vi "Emit.vi"(6 "inparameter":variant, 8 "error in (no error)":errorcluster, 9 "parameter":variant, 10 "function":string, 11 "output in":refnum<class "Output.lvclass">) -> (0 "error out":errorcluster, 3 "output out":refnum<class "Output.lvclass">)   [LabVIEW 2015, in "Output.lvclass"]
uses:
  Output.lvclass
  Output.lvclass/Output.ctl
  <vilib>/addons/lv-msgpack/MsgPack Serializer/MsgPackSerializer.lvclass
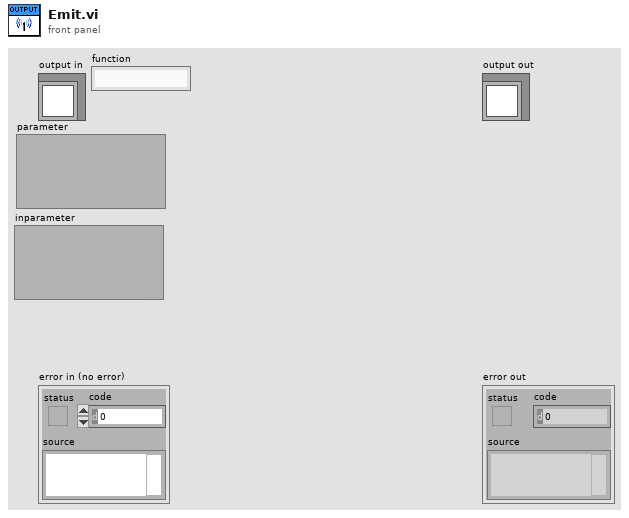
[diagram p1: front panel]
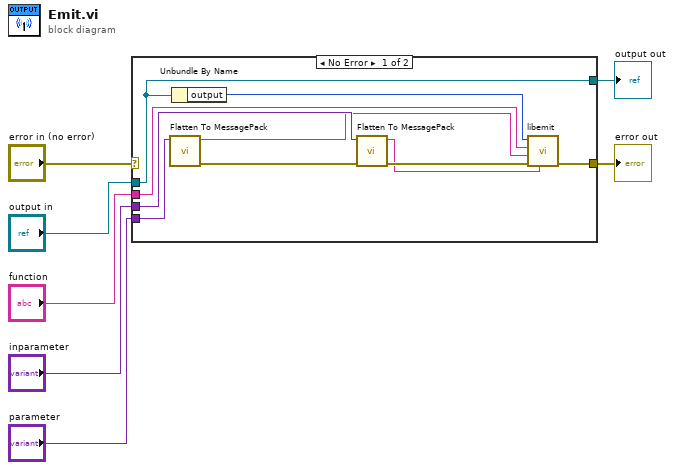
[diagram p0: block diagram]
diagram:
  n1 = case shown="No Error" "error in (no error)" {
    selector: "error in (no error)" -> [_ w19]
    tunnel: [w10 w19] -> w6
    tunnel: [w8 w18] -> w4
    tunnel: "output in" -> [w8 w18]
    tunnel: "parameter" -> [w17 _]
    tunnel: "inparameter" -> [w15 _]
    tunnel: "function" -> [w13 _]
    frame No Error {
      n2 = call <vilib>:"Flatten To MessagePack.vi"("Data"=w17) -> ("error out"=w16:errorcluster, "MsgPack Data"=w14:string)  [unwired: 9 in]
      n3 = Unbundle By Name(w8) -> ("output"=w9:i32)
      n4 = call <vilib>:"Flatten To MessagePack.vi"("error in (no error)"=w16, "Data"=w15) -> ("error out"=w12:errorcluster, "MsgPack Data"=w11:string)  [unwired: 8 in]
      n5 = call "libemit.vi"("inparams"=w11, "error in (no error)"=w12, "parameter"=w14, "function"=w13, "output"=w9) -> ("error out"=w10:errorcluster)  [unwired: 6 in]
    }
    frame Error {
    }
  }
  "error out" <- w6
  "output out" <- w4
